vi "TP 3.2.vi"() -> ()   [LabVIEW 2013]
uses:
  <vilib>/sound2/lvsound2.llb/Sound Output Write (DBL).vi
panel:
  in  "Cluster":T1
  in  "Stop":bool
  out "Waveform Graph":dbl[][](graph)
  in  "Amplitud":dbl=6.0
  in  "Frecuencia":dbl=10.0
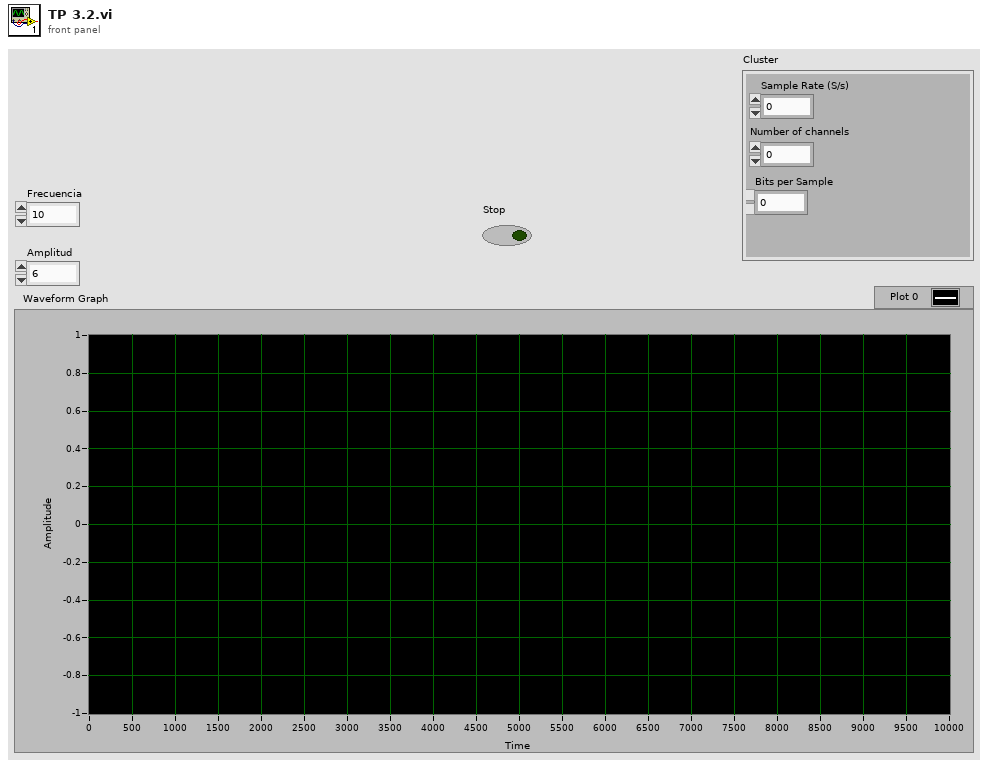
[diagram p1: front panel]
types:
  T1 = cluster{"Sample Rate (S/s)":dbl, "Number of channels":i32, "Bits per Sample":i32}
  T2 = typedef "Sound Output Task ID.ctl" = u32
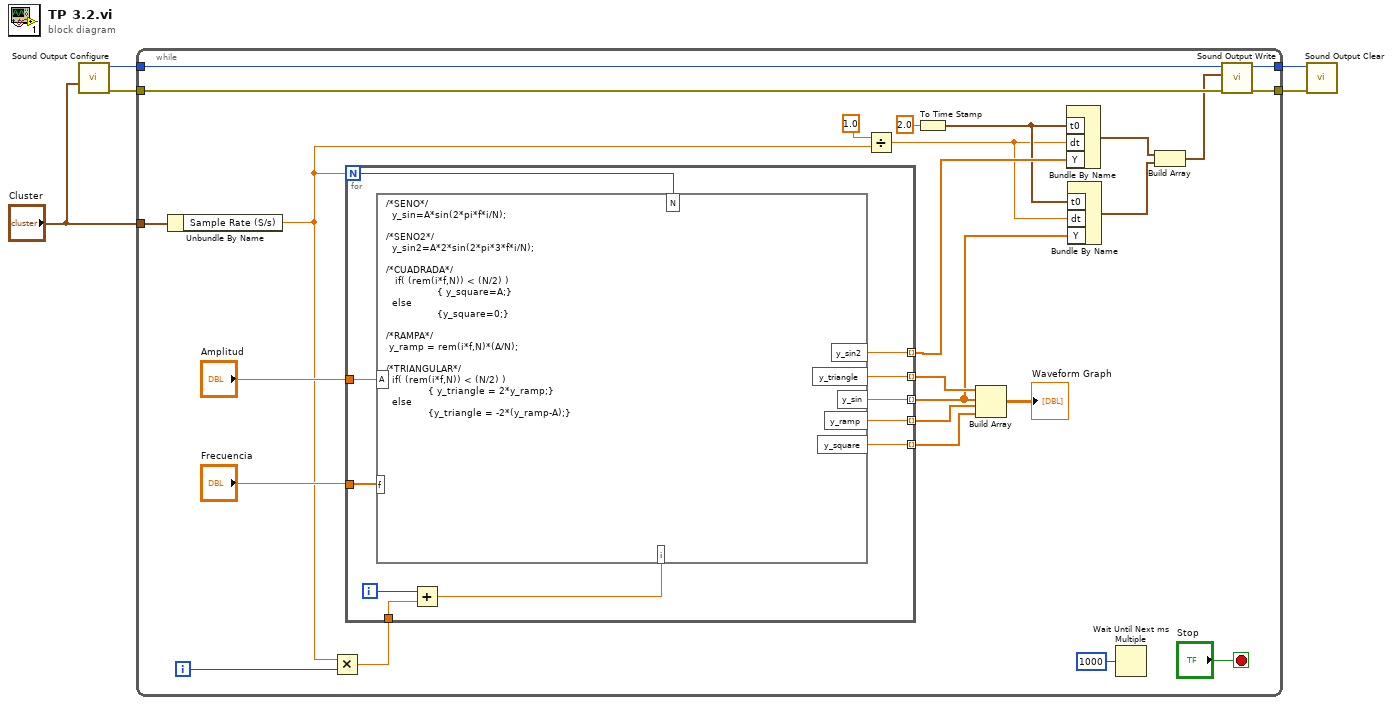
[diagram p0: block diagram]
diagram:
  n1 = call <vilib>:"Sound Output Configure.vi"("sound format"="Cluster") -> ("error out"=w1:errorcluster, "task ID"=w2:T2)  [unwired: 9 in]
  n2 = while {
    tunnel: "Cluster" -> [w20]
    tunnel: [w19] -> w4
    tunnel: [w18] -> w3
    tunnel: w2 -> [w14]
    tunnel: w1 -> [w12]
    i -> [w29]
    stop <- "Stop" stop-if-true
    n3 = Unbundle By Name(w20) -> ("Sample Rate (S/s)"=w13:dbl)
    n4 = Multiply(x=w13, y=w29) -> (x*y=w28:dbl)
    n5 = for {
      N: w13 -> [w32]
      tunnel: "Frecuencia" -> [w33]
      tunnel: [w41] -> w15 mode=indexing
      tunnel: w28 -> [w34]
      tunnel: [w39] -> w24 mode=indexing
      tunnel: [w38] -> w23 mode=indexing
      tunnel: [w37] -> w22 mode=indexing
      tunnel: "Amplitud" -> [w36]
      tunnel: [w31] -> w16 mode=indexing
      i -> [w35]
      n6 = Add(x=w35, y=w34) -> (x+y=w40:dbl)
      n7 = formula code="/*SENO*/\n  y_sin=A*sin(2*pi*f*i/N);\n\n/*SENO2*/\n  y_sin2=A*2*sin(2*pi*3*f*i/N);\n\n/*CUADRADA*/\n   if( (rem(i*f,N)) < (N/2) )\n                 { y_square=A;}\n  else\n                 {y_square=0;}\n\n/*RAMPA*/\n y_ramp = rem(i*f,N)*(A/N);\n\n/*TRIANGULAR*/\n  if( (rem(i*f,N)) < (N/2) )\n              { y_triangle = 2*y_ramp;}\n  else\n              {y_triangle = -2*(y_ramp-A);}"("A"=w36, "N"=w32, "i"=w40, "f"=w33) -> ("y_sin"=w41:dbl, "y_ramp"=w38:dbl, "y_square"=w37:dbl, "y_triangle"=w39:dbl, "y_sin2"=w31:dbl)
    }
    n8 = Divide(x=1.0, y=w13) -> (x/y=w8:dbl)
    n9 = To Time Stamp(1:2.0) -> (0:w9:timestamp)
    n10 = Build Array(w24, w15, w23, w22) -> (→"Waveform Graph":dbl[][])
    n11 = Bundle By Name ("Build Waveform")("t0"=w9, "dt"=w8, "Y"=w16) -> (w10:waveform(dbl))  [unwired: 1 in]
    n12 = Bundle By Name ("Build Waveform")("t0"=w9, "dt"=w8, "Y"=w15) -> (w7:waveform(dbl))  [unwired: 1 in]
    n13 = Wait Until Next ms Multiple(millisecond multiple=u32 1000) -> ()  [unwired: 1 out]
    n14 = Build Array(w10, w7) -> (w11:waveform(dbl)[])
    n15 = call-poly <vilib>:"Sound Output Write.vi"("error in (no error)"=w12, "data"=w11, "task ID"=w14) -> ("error out"=w19:errorcluster, "task ID out"=w18:T2)  [unwired: 7 in]
  }
  n16 = call <vilib>:"Sound Output Clear.vi"("error in (no error)"=w4, "task ID"=w3) -> ()  [unwired: 9 in, 1 out]
